vi "A12rowmm.vi"(0 "Basic Size":dbl, 5 "error in":errorcluster) -> (6 "Row":dbl, 8 "error out":errorcluster)   [LabVIEW 2023]
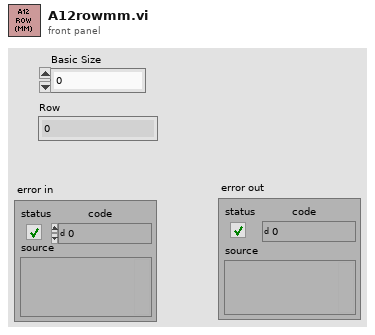
[diagram p1: front panel]
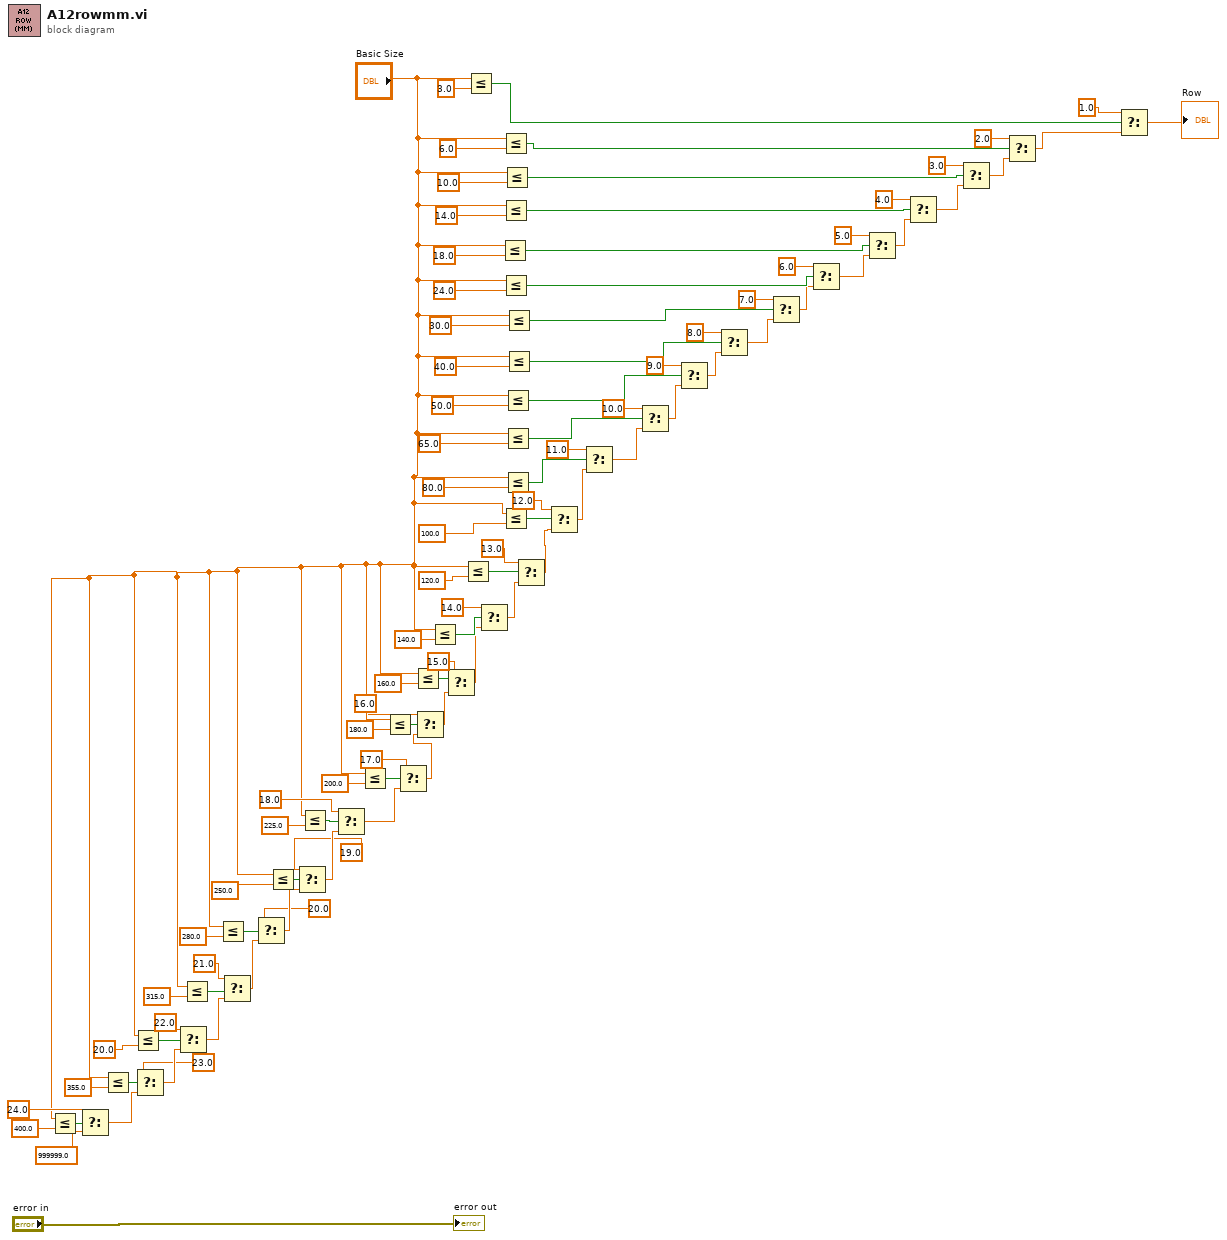
[diagram p0: block diagram]
diagram:
  n1 = Less Or Equal?(x="Basic Size", y=400.0) -> (x <= y?=w7:bool)
  n2 = Select(t=24.0, s=w7, f=999999.0) -> (s? t:f=w9:dbl)
  n3 = Less Or Equal?(x="Basic Size", y=355.0) -> (x <= y?=w12:bool)
  n4 = Less Or Equal?(x="Basic Size", y=20.0 ("t")) -> (x <= y?=w16:bool)
  n5 = Select(t=23.0, s=w12, f=w9) -> (s? t:f=w13:dbl)
  n6 = Select(t=22.0, s=w16, f=w13) -> (s? t:f=w17:dbl)
  n7 = Less Or Equal?(x="Basic Size", y=315.0) -> (x <= y?=w20:bool)
  n8 = Less Or Equal?(x="Basic Size", y=280.0) -> (x <= y?=w24:bool)
  n9 = Select(t=21.0, s=w20, f=w17) -> (s? t:f=w21:dbl)
  n10 = Select(t=20.0, s=w24, f=w21) -> (s? t:f=w25:dbl)
  n11 = Less Or Equal?(x="Basic Size", y=250.0) -> (x <= y?=w28:bool)
  n12 = Select(t=19.0, s=w28, f=w25) -> (s? t:f=w29:dbl)
  n13 = Less Or Equal?(x="Basic Size", y=225.0) -> (x <= y?=w32:bool)
  n14 = Select(t=18.0, s=w32, f=w29) -> (s? t:f=w33:dbl)
  n15 = Less Or Equal?(x="Basic Size", y=200.0) -> (x <= y?=w35:bool)
  n16 = Less Or Equal?(x="Basic Size", y=180.0) -> (x <= y?=w38:bool)
  n17 = Select(t=17.0, s=w35, f=w33) -> (s? t:f=w36:dbl)
  n18 = Less Or Equal?(x="Basic Size", y=160.0) -> (x <= y?=w42:bool)
  n19 = Select(t=16.0, s=w38, f=w36) -> (s? t:f=w39:dbl)
  n20 = Less Or Equal?(x="Basic Size", y=140.0) -> (x <= y?=w45:bool)
  n21 = Select(t=15.0, s=w42, f=w39) -> (s? t:f=w43:dbl)
  n22 = Less Or Equal?(x="Basic Size", y=120.0) -> (x <= y?=w51:bool)
  n23 = Less Or Equal?(x="Basic Size", y=3.0) -> (x <= y?=w98:bool)
  n24 = Select(t=14.0, s=w45, f=w43) -> (s? t:f=w47:dbl)
  n25 = Less Or Equal?(x="Basic Size", y=18.0) -> (x <= y?=w82:bool)
  n26 = Less Or Equal?(x="Basic Size", y=6.0) -> (x <= y?=w94:bool)
  n27 = Less Or Equal?(x="Basic Size", y=14.0) -> (x <= y?=w86:bool)
  n28 = Less Or Equal?(x="Basic Size", y=24.0) -> (x <= y?=w78:bool)
  n29 = Less Or Equal?(x="Basic Size", y=100.0 ("x")) -> (x <= y?=w56:bool)
  n30 = Less Or Equal?(x="Basic Size", y=10.0) -> (x <= y?=w91:bool)
  n31 = Less Or Equal?(x="Basic Size", y=50.0) -> (x <= y?=w66:bool)
  n32 = Less Or Equal?(x="Basic Size", y=65.0) -> (x <= y?=w62:bool)
  n33 = Less Or Equal?(x="Basic Size", y=80.0) -> (x <= y?=w58:bool)
  n34 = Less Or Equal?(x="Basic Size", y=30.0) -> (x <= y?=w74:bool)
  n35 = Less Or Equal?(x="Basic Size", y=40.0) -> (x <= y?=w70:bool)
  n36 = Select(t=13.0, s=w51, f=w47) -> (s? t:f=w50:dbl)
  n37 = Select(t=12.0, s=w56, f=w50) -> (s? t:f=w55:dbl)
  n38 = Select(t=11.0, s=w58, f=w55) -> (s? t:f=w60:dbl)
  n39 = Select(t=10.0, s=w62, f=w60) -> (s? t:f=w65:dbl)
  n40 = Select(t=9.0, s=w66, f=w65) -> (s? t:f=w68:dbl)
  n41 = Select(t=8.0, s=w70, f=w68) -> (s? t:f=w72:dbl)
  n42 = Select(t=7.0, s=w74, f=w72) -> (s? t:f=w76:dbl)
  n43 = Select(t=6.0, s=w78, f=w76) -> (s? t:f=w80:dbl)
  n44 = Select(t=5.0, s=w82, f=w80) -> (s? t:f=w84:dbl)
  n45 = Select(t=4.0, s=w86, f=w84) -> (s? t:f=w88:dbl)
  n46 = Select(t=3.0, s=w91, f=w88) -> (s? t:f=w92:dbl)
  n47 = Select(t=2.0, s=w94, f=w92) -> (s? t:f=w95:dbl)
  n48 = Select(t=1.0, s=w98, f=w95) -> (s? t:f=→"Row":dbl)
  "error out" <- "error in"
